vi "Customize Ctrls.vi"(8 "error in (no error)":errorcluster, 9 "Permission Labels Ref":refnum<vi>, 10 "Array Element Ref":refnum<vi>, 11 "Mode":string) -> (0 "error out":errorcluster)   [LabVIEW 2016, in "UserPwd DB.lvlib" / "UserPwd DB Configuration.lvclass"]
uses:
  <userlib>/Common Components/UserPwd DB/UserPwd DB Config/UserPwd DB Configuration.lvclass
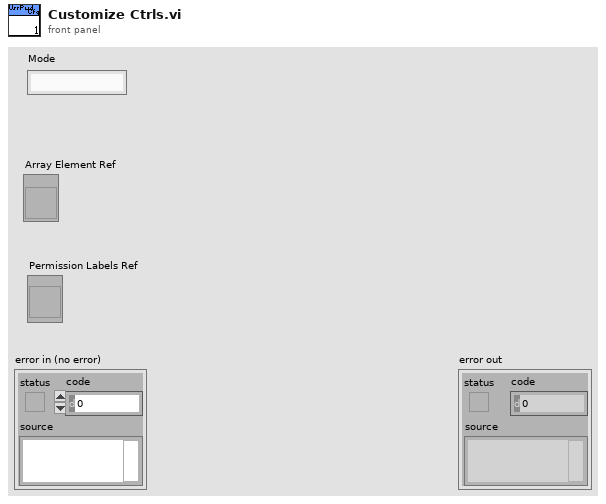
[diagram p1: front panel]
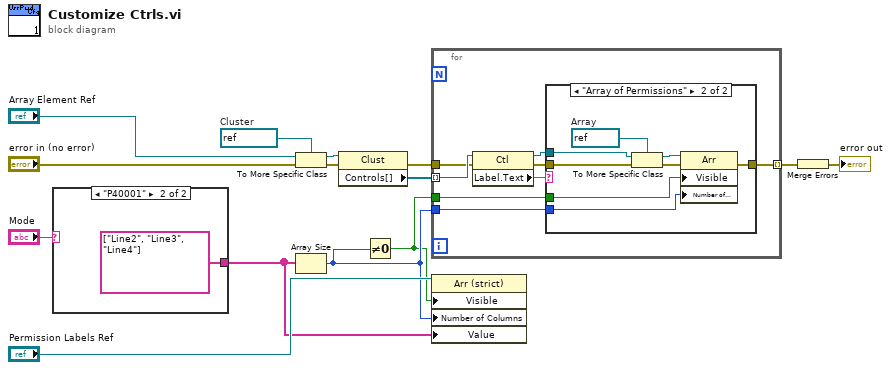
[diagram p0: block diagram]
diagram:
  w13 = refnum<vi> refnum  # Cluster
  n1 = case shown="\"P40001\"" "Mode" {
    tunnel: [_ string[] ["Line2", "Line3", "Line4"] ("Permission Labels")] -> w4
    frame Default {
    }
    frame "P40001" {
    }
  }
  n2 = To More Specific Class(target class=w13, reference="Array Element Ref", error in="error in (no error)") -> (specific class reference=w12:refnum<vi>, error out=w10:errorcluster)
  n3 = Array Size(array=w4) -> (size(s)=w3:i32)
  n4 = property class="Clust"(reference=w12, error in=w10) -> (error out=w8:errorcluster, "Controls[]"=w9:refnum<vi>[])  [unwired: 1 out]
  n5 = Not Equal To 0?(x=w3) -> (x != 0?=w2:bool)
  n6 = for {
    tunnel: w9 -> [w23] mode=indexing
    tunnel: w8 -> [w21]
    tunnel: w3 -> [w18]
    tunnel: [w17] -> w7 mode=indexing
    tunnel: w2 -> [w16]
    n7 = property class="Ctl"(reference=w23, error in=w21) -> (reference out=w19:refnum<vi>, error out=w20:errorcluster, "Label.Text"=w22:string)
    n8 = case shown="\"Array of Permissions\"" w22 {
      tunnel: w20 -> [w24 w32]
      tunnel: w19 -> [_ w31]
      tunnel: w18 -> [_ w28]
      tunnel: [w24 w26] -> w17
      tunnel: w16 -> [_ w25]
      frame Default {
      }
      frame "Array of Permissions" {
        w30 = refnum<vi> refnum  # Array
        n9 = To More Specific Class(target class=w30, reference=w31, error in=w32) -> (specific class reference=w29:refnum<vi>, error out=w27:errorcluster)
        n10 = property class="Arr"(reference=w29, error in=w27, "Visible"=w25, "Number of Columns"=w28) -> (error out=w26:errorcluster)  [unwired: 1 out]
      }
    }
  }
  n11 = property class="Arr (strict)"(reference="Permission Labels Ref", "Visible"=w2, "Number of Columns"=w3, "Value"=w4) -> ()  [unwired: 1 in, 2 out]
  n12 = Merge Errors(w7) -> (→"error out":errorcluster)
